vi "Get 2D Array Element.vi"(8 "error in (no error)":errorcluster, 9 "Col":i32, 10 "Row":i32, 11 "Array":string[][](array[string])) -> (0 "error out":errorcluster, 2 "String":string, 3 "Array Out":string[][](array[string]))   [LabVIEW 2015]
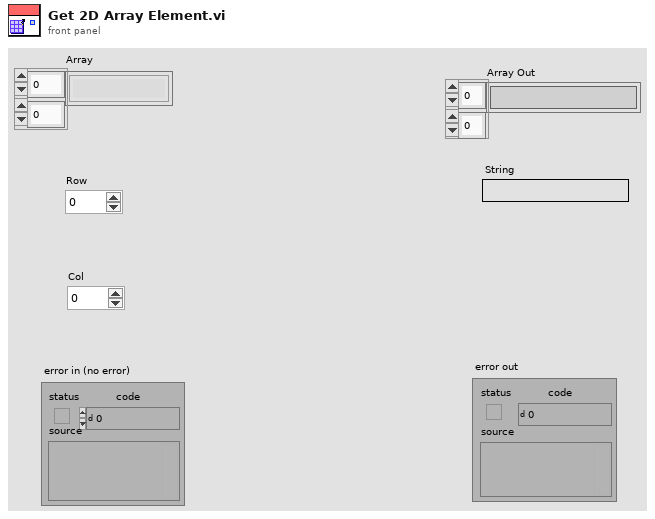
[diagram p1: front panel]
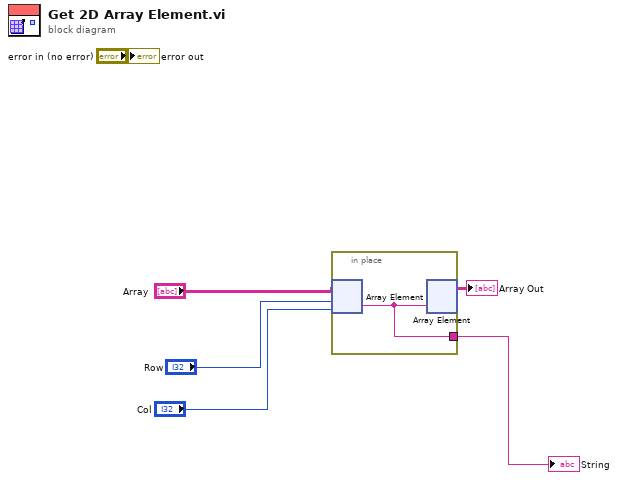
[diagram p0: block diagram]
diagram:
  n1 = in-place {
    in-place-border: [w6] -> w4
    n2 = in-place-array #1("Array", "Row", "Col") -> (w6:string)
    n3 = in-place-array #1(w6) -> (→"Array Out":string[][])  [unwired: 2 out]
  }
  "String" <- w4
